vi "ScheduledExitMessage_Parse.vi"(8 "error in (no error)":errorcluster, 11 "scheduled exit message":variant) -> (0 "error out":errorcluster, 3 "scheduled exit reason":string)   [LabVIEW 2017, in "Controller.lvlib"]
uses:
  <vilib>/addons/InsightCM/Devices/Shared/Common/Controller/Controller.lvlib
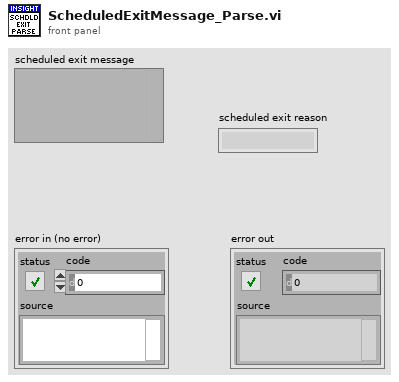
[diagram p1: front panel]
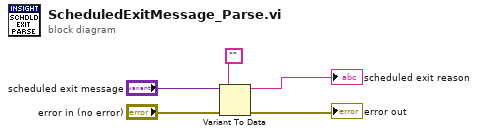
[diagram p0: block diagram]
diagram:
  n1 = Variant To Data(error in="error in (no error)", type="", Variant="scheduled exit message") -> (data=→"scheduled exit reason":string, error out=→"error out":errorcluster)
